vi "MCU_ReadTemp.vi"(8 "error in (no error)":errorcluster, 11 "VISA resource name":refnum<visa-resource-name>) -> (0 "error out":errorcluster, 3 "Volt":dbl[](array[numeric]))   [LabVIEW 2018, in "Acquire Data.lvclass"]
uses:
  Acquire Data.lvclass
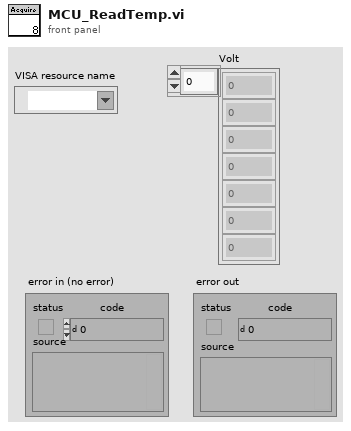
[diagram p1: front panel]
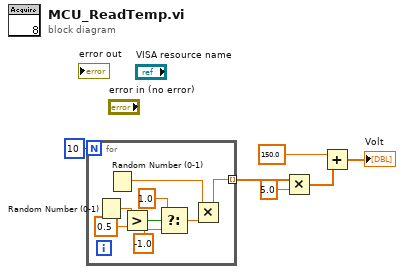
[diagram p0: block diagram]
diagram:
  n1 = for {
    N: 10 -> [_]
    tunnel: [w7] -> w3 mode=indexing
    n2 = Random Number (0-1)() -> (number: 0 to 1=w14:dbl)
    n3 = Random Number (0-1)() -> (number: 0 to 1=w8:dbl)
    n4 = Greater?(x=w14, y=0.5) -> (0:w12:bool)
    n5 = Select(t=1.0, s=w12, f=-1.0 ("t")) -> (s? t:f=w9:dbl)
    n6 = Multiply(x=w8, y=w9) -> (x*y=w7:dbl)
  }
  n7 = Multiply(x=w3, y=5.0) -> (x*y=w1:dbl[])
  n8 = Add(x=150.0, y=w1) -> (x+y=→"Volt":dbl[])
